vi "AM_PID_tester_2.vi"() -> ()   [LabVIEW 2013]
uses:
  DataMode.ctl
  Input_5782/5782_states.ctl
  <vilib>/Platform/TimedLoop/XDataNode/timing_clust.ctl
  <vilib>/Platform/TimedLoop/XDataNode/nitl_modes.ctl
  <vilib>/Platform/TimedLoop/XDataNode/wakeup.ctl
  <vilib>/rvi/FXPMathLib/FxpConvert/subVIs/nifxpmath_Convert_SimConfig.ctl
  <vilib>/fxp/LVFixedPointQuantizationPolicyTypeDef.ctl
  <vilib>/fxp/LVFixedPointOverflowPolicyTypeDef.ctl
  <vilib>/rvi/Emulation/niFpgaSctlEmulationGetInTimedLoop.vi
  <vilib>/rvi/Emulation/niFpgaEmulationReportErrorSimple.vi
  <vilib>/rvi/Emulation/niFpgaGetClockAttributes.vi
  <vilib>/rvi/eio/common/nirviEmuTemplateMethod_errors.vi
  <vilib>/rvi/Emulation/niFpgaCriticalErrorInLSC.vi
  <vilib>/rvi/DataTransferAndStorage/Register/Emulation/niFpgaRegisterEmulationFpgaImpl.vi
  <instcachedir>/0/niFpgaRegisterEmulationFpgaImpl_DCF4BC0110594B98B44A971D60CEEC4D.lvgen/niFpgaRegisterEmulationFpgaImpl_DCF4BC0110594B98B44A971D60CEEC4D_005.vi
  <vilib>/rvi/DataTransferAndStorage/Container/Common/niFpgaContainerGetUniqueNameForEmu.vi
  <instcachedir>/0/niFpgaRegisterEmulationFpgaImpl_DCF4BC0110594B98B44A971D60CEEC4D.lvgen/niFpgaRegisterEmulationFpgaImpl_DCF4BC0110594B98B44A971D60CEEC4D_016.vi
  <instcachedir>/0/niFpgaRegisterEmulationFpgaImpl_DCF4BC0110594B98B44A971D60CEEC4D.lvgen/niFpgaRegisterEmulationFpgaImpl_DCF4BC0110594B98B44A971D60CEEC4D_017.vi
  <instcachedir>/0/niFpgaRegisterEmulationFpgaImpl_DCF4BC0110594B98B44A971D60CEEC4D.lvgen/niFpgaRegisterEmulationFpgaImpl_DCF4BC0110594B98B44A971D60CEEC4D_012.vi
  <instcachedir>/0/niFpgaRegisterEmulationFpgaImpl_DCF4BC0110594B98B44A971D60CEEC4D.lvgen/niFpgaRegisterEmulationFpgaImpl_DCF4BC0110594B98B44A971D60CEEC4D_015.vi
  <vilib>/rvi/FIFO/Fifo_Resource/nirvififoEmulationReadFpgaImpl.vi
  <vilib>/rvi/interface/RandomDataEmulation/nirviRandomDataMultiElementFPGAFIFO.vi
  <instcachedir>/0/nirviRandomDataMultiElementFPGAFIFO_F2B80EDE0D7944A08478D8D26097D4DB.lvgen/nirviRandomDataMultiElementFPGAFIFO_F2B80EDE0D7944A08478D8D26097D4DB_005.vi
  <vilib>/rvi/interface/RandomDataEmulation/niFpgaRandomDataHandleErrors.vi
  <instcachedir>/0/niFpgaRegisterEmulationFpgaImpl_DCF4BC0110594B98B44A971D60CEEC4D.lvgen/niFpgaRegisterEmulationFpgaImpl_DCF4BC0110594B98B44A971D60CEEC4D_009.vi
  <vilib>/rvi/interface/RandomDataEmulation/nirviRandomDataFPGAFIFO.vi
  <vilib>/rvi/FXPMathLib/FxpConvert/simVIs/DllFxpConvertTemp_sub.vi
  <vilib>/rvi/FIFO/Fifo_Resource/nirvififoEmulationWriteFpgaImpl.vi
  <vilib>/Platform/TimedLoop/XDataNode/XDataNode.xnode
  <vilib>/eio/EIONode/EIONode.xnode
  <vilib>/rvi/DataTransferAndStorage/Container/XNode/niFpgaContainer.xnode
  <vilib>/rvi/DataTransferAndStorage/Register/Emulation/niFpgaRegisterEmulation.vi
  <vilib>/rvi/FIFO/Fifo_Resource/nirvififoEmulationRead.vi
  <vilib>/rvi/interface/RandomDataEmulation/nirviRandomDataFpgaMultiElementTemplate.vi
  <vilib>/rvi/interface/RandomDataEmulation/nirviRandomDataFpgaReadWriteTemplate.vi
  <vilib>/rvi/FXPMathLib/FxpInterpret/XNode/nifxpmath_Interpret.xnode
  <vilib>/rvi/FXPMathLib/FxpConvert/XNode/nifxpmath_Convert.xnode
  <vilib>/rvi/FIFO/Fifo_Resource/nirvififoEmulationWrite.vi
  <vilib>/rvi/FXPMathLib/FxpSub/XNode/nifxpmath_Sub.xnode
  <vilib>/Platform/TimedLoop/XDataNode/XDNodeRunTimeDep.lvlib
  <vilib>/rvi/FXPMathLib/sim/FxpSim.dll
panel:
  in  "AM phase":fxp<+,64,64>
  in  "Continuous":bool
  in  "Downsample":fxp<+,8,8>=1.0
  in  "new coeffs":bool
  in  "FIR coeffs":fxp<+/-,18,18>[](array[numeric])
  in  "CIC Gain":fxp<+/-,32,1>=0.00390625 format="%#_32g"
  in  "Acquisition running":bool
  in  "Phase output":fxp<+,64,64>[](array[numeric])=[0.0, 0.0, 0.0, 0.0, 0.0, 0.0, 0.0, 0.0]
  in  "Simulated phase 5782":fxp<+,64,64>[](array[numeric])=[0.0, 0.0]
  in  "Mode":T1
  in  "Phase 5782":fxp<+,64,64>[](array[numeric])=[0.0, 0.0]
  out "IO Module\\Trigger Input":bool
  in  "IO Module\\AO Data Sync":bool=TRUE
  in  "IO Module\\SPI Write Data":u16
  out "IO Module\\SPI Read Data":u8
  in  "IO Module\\SPI Read":bool
  in  "IO Module\\SPI Write":bool
  in  "IO Module\\SPI Address":u16
  in  "IO Module\\SPI Device":u8
  out "IO Module\\SPI Idle":bool
  in  "delay phase":fxp<+,64,64>
  in  "User Command Commit":bool
  in  "User Command":u8
  out "User Command Idle":bool
  out "User Command Status":u8
  in  "User Data 0":u8
  in  "User Data 1":u8
  out "PLL Locked":bool
  out "User Error":bool
  out "Configured?":bool
  in  "5782 record length":u16=4000 caption="Samples Per Trigger" min=1 step=1
  in  "Trigger Acquisition":bool
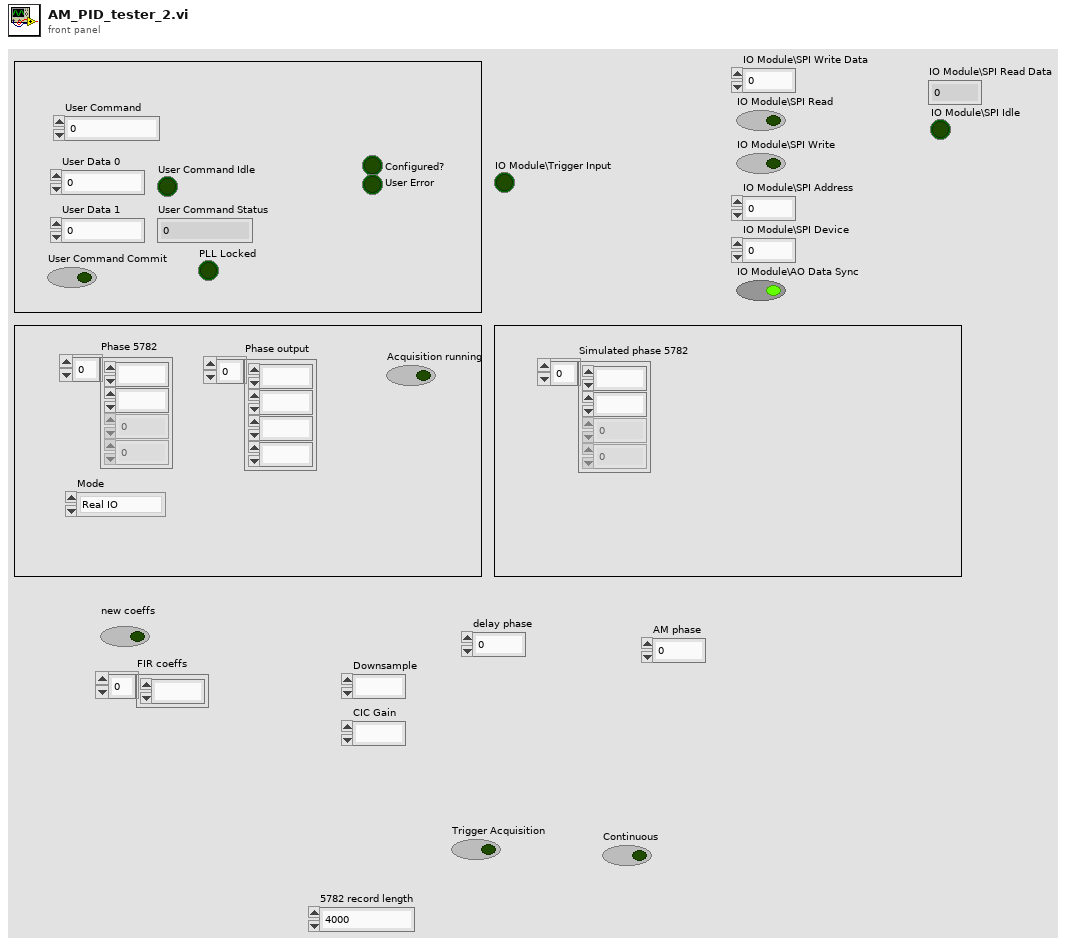
[diagram p1: front panel]
types:
  T1 = typedef "DataMode.ctl" = enum16{"Real IO", "Simulated"}
  T2 = typedef "5782_states.ctl" = enum8{"Wait for trigger", "Acquisition", "Send record length", "Quiet period"}
  T3 = typedef "XDNodeRunTimeDep.lvlib/timing_clust.ctl" = cluster{"Expected End [f-1]":u64, "Actual End [f-1]":u64, "Finished Late? [f-1]":bool, "Expected End [i-1]":u64, "Actual End [i-1]":u64, "Finished Late? [i-1]":bool, "Expected Start [i]":u64, "Actual Start [i]":u64, "Expected Start [f]":u64, "Actual Start [f]":u64, "Source Name":string, "Structure Name":string, "Period":i64, "Deadline":i64, "Offset":i64, "Start":i64, "Priority":i32, "Timeout":i32, "Mode":T4, "Wakeup Reason":T5, "Error":errorcluster, "Source Type":string, "Secondary Source Type":string, "Global End Time":u64, "Global Start Time":u64, "Frame Duration":u64, "Iteration Duration":u64, "Assigned CPU":i32, "I/O Scan Engine Mode":u32}
  T4 = typedef "XDNodeRunTimeDep.lvlib/nitl_modes.ctl" = enum32{"No Change", "Process missed periods, maintain original phase", "Discard missed periods, maintain original phase", "Process missed periods, ignore original phase", "Discard missed periods, ignore original phase"}
  T5 = typedef "XDNodeRunTimeDep.lvlib/wakeup.ctl" = enum32{"Normal", "Aborted", "Asynchronous wakeup", "Timing source error", "Timed loop error", "Timeout"}
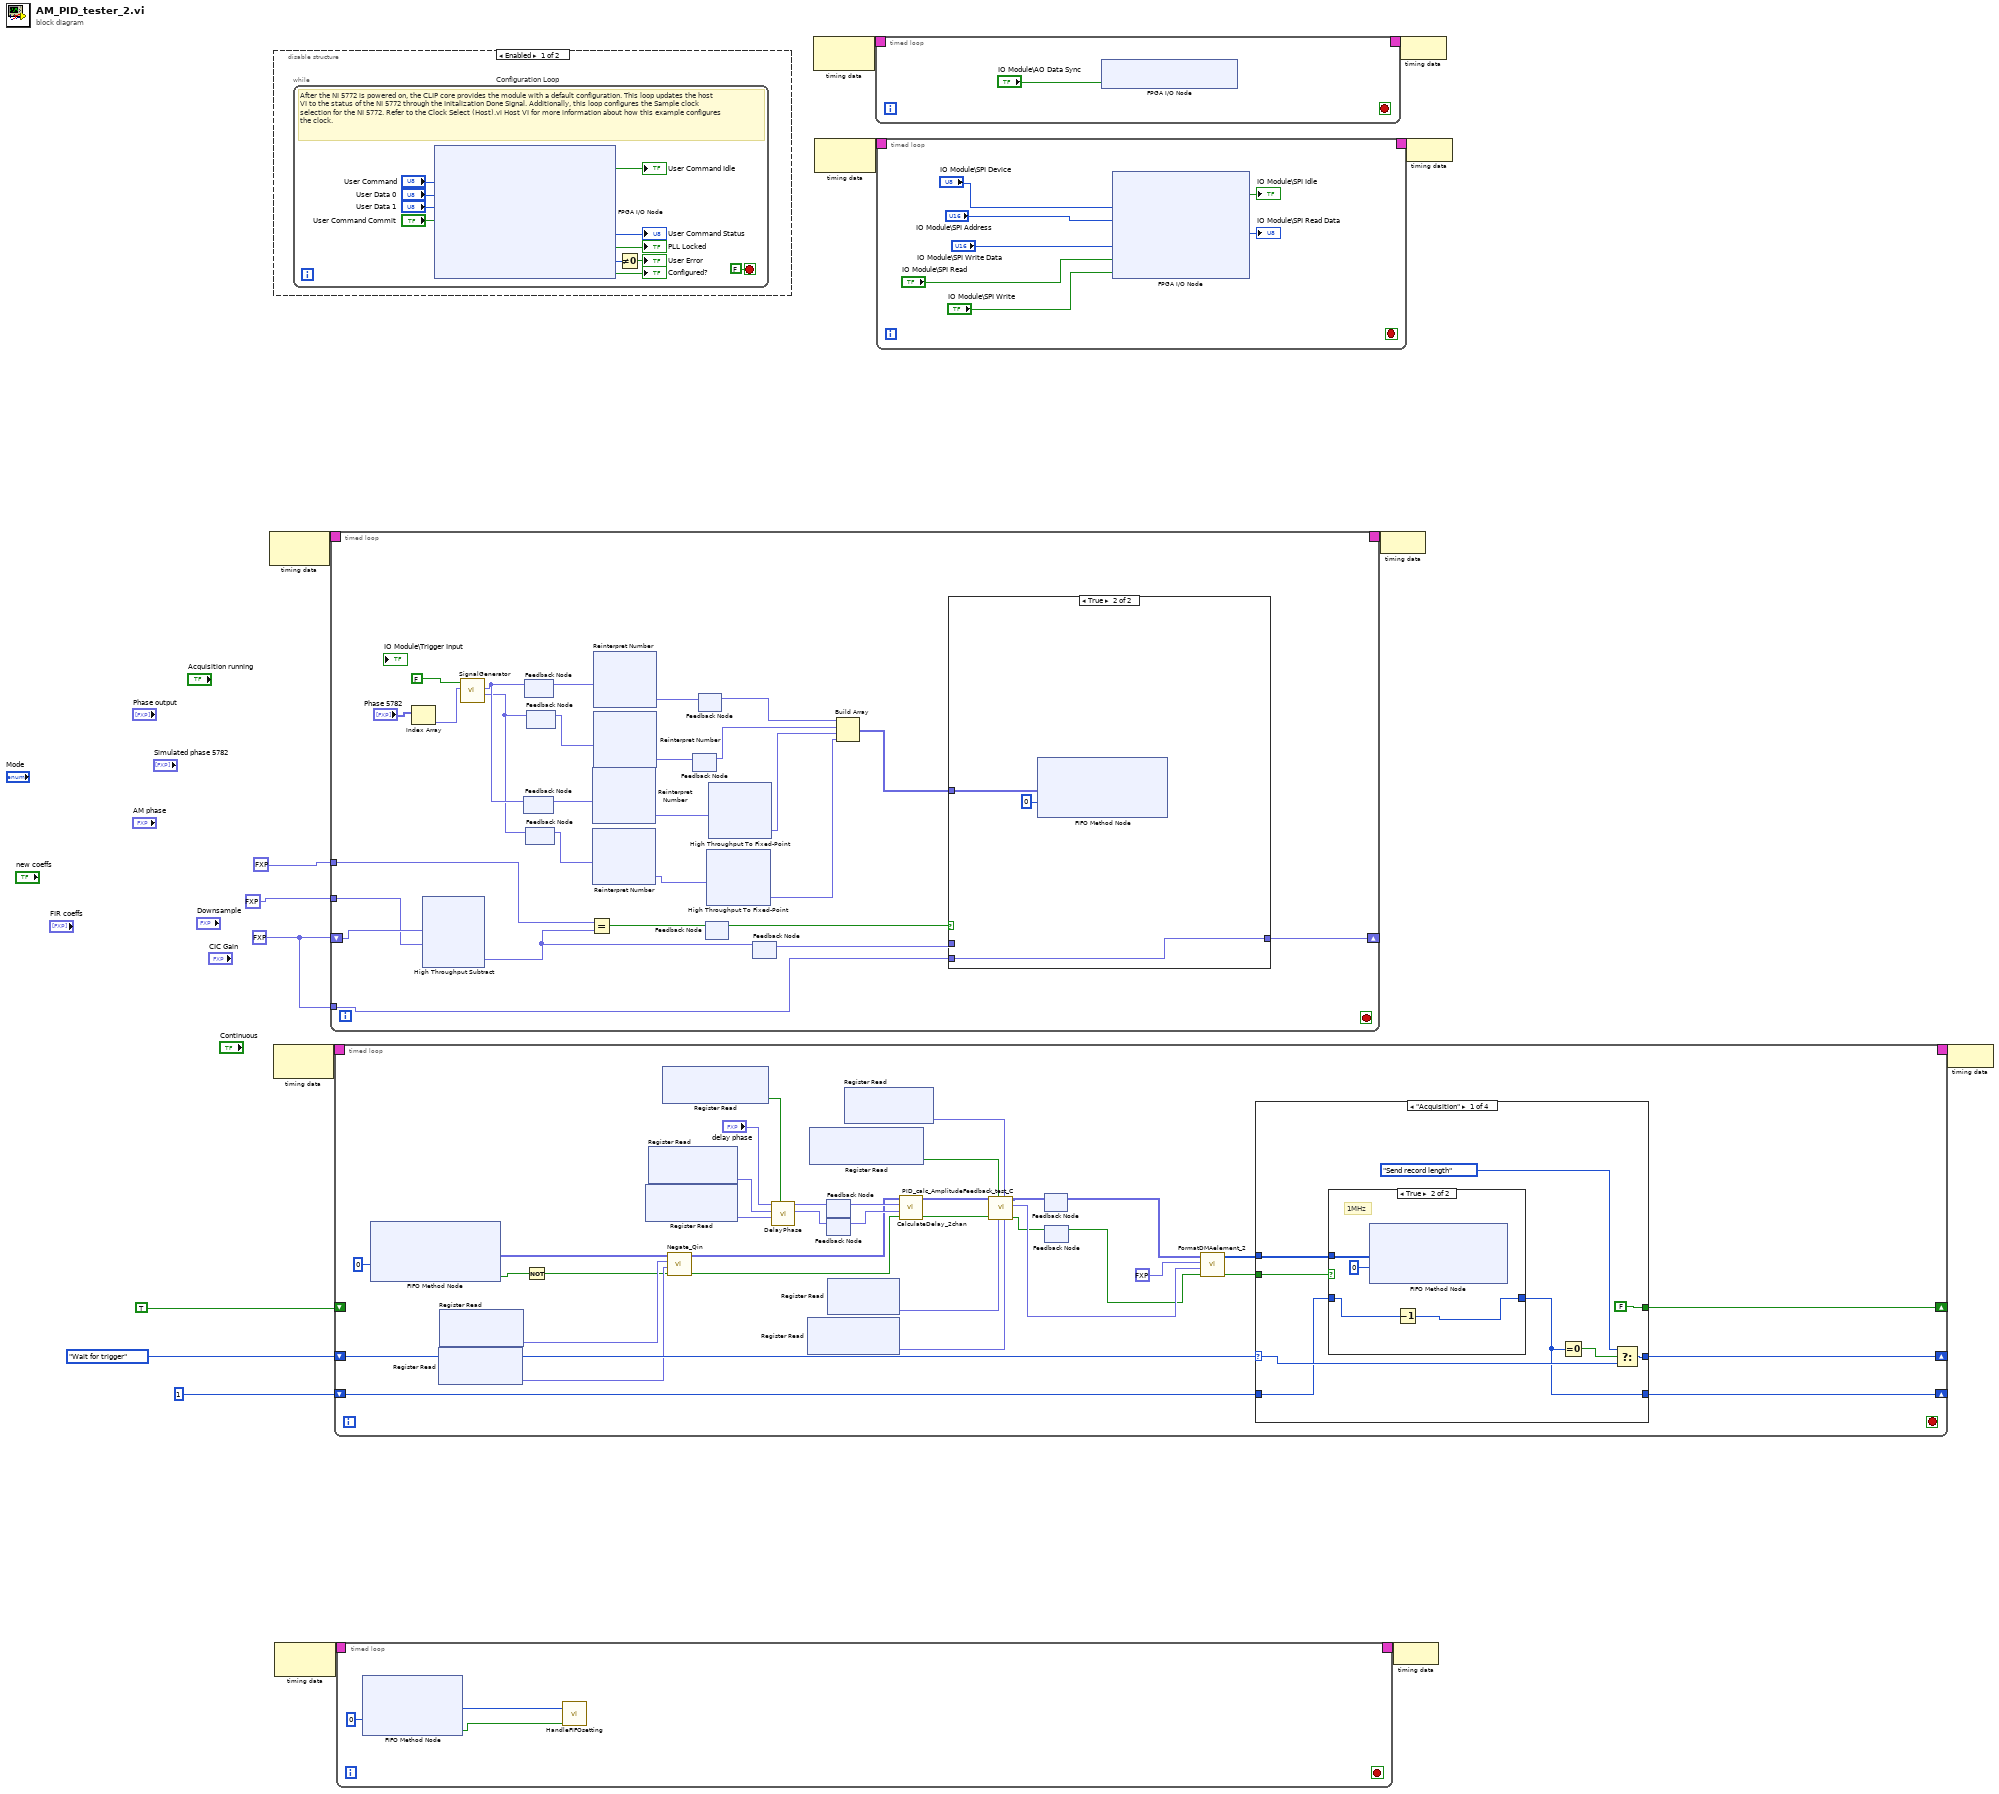
[diagram p0: block diagram]
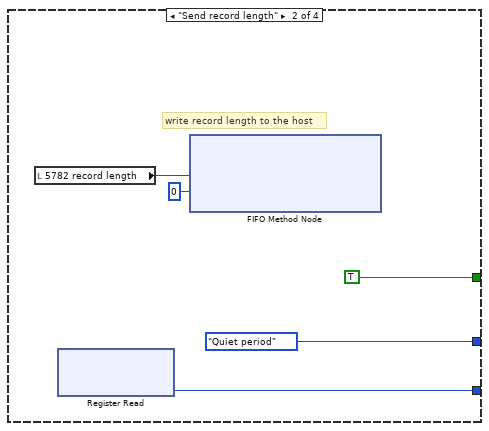
[diagram p4: hidden frame]
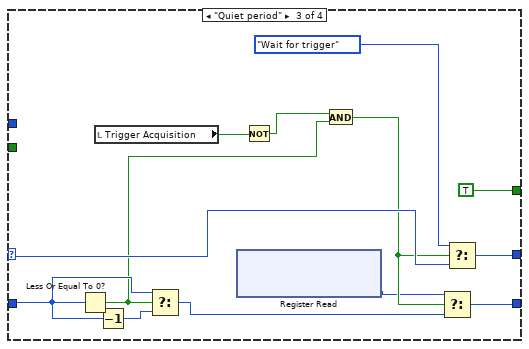
[diagram p5: hidden frame]
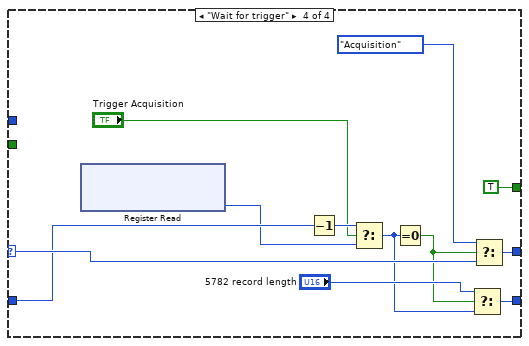
[diagram p6: hidden frame]
diagram:
  w3 = fxp<+/-,8,8> 5.0 ("x")
  n1 = node-c288() -> (w2:T3)  [unwired: 1 in]
  n2 = disable-structure shown="Enabled" {
    frame Enabled {
      n3 = while "Configuration Loop" {
        stop <- FALSE stop-if-true
        # "After the NI 5772 is powered on, the CLIP core provides the module with a default configuration. This loop updates the host VI to the status of the NI 5772 through the Initalization Done Signal. Additionally, this loop configures the Sample clock selection for the NI 5772. Refer to the Clock Select (Host).vi Host VI for more information about how this example configures the clock."
        n4 = xnode "FPGA I/O Node"("IO Module\\User Command"="User Command", "IO Module\\User Data 0"="User Data 0", "IO Module\\User Data 1"="User Data 1", "IO Module\\User Command Commit"="User Command Commit") -> ("IO Module\\User Command Idle"=→"User Command Idle":bool, "IO Module\\User Command Status"=→"User Command Status":u8, "IO Module\\PLL Locked"=→"PLL Locked":bool, "IO Module\\User Error"=w22:u8, "IO Module\\Initialization Done"=→"Configured?":bool)  [unwired: 9 in, 9 out]
        n5 = Not Equal To 0?(x=w22) -> (x != 0?=→"User Error":bool)
      }
    }
    frame Disabled {
    }
  }
  n6 = node-c288() -> (w16:T3)  [unwired: 1 in]
  n7 = node-c288() -> (w11:T3)  [unwired: 1 in]
  n8 = timed-loop {
    shift-right: [w50] -> _
    shift-left: w3 -> [w54]
    tunnel: fxp<+/-,8,8> 1.0 ("y") -> [w53]
    tunnel: fxp<+/-,8,8> 0.0 ("y") -> [w52]
    tunnel: w3 -> [w51]
    timing: w2 -> [_]
    timing-out: [_] -> w1
    stop <- _ stop-if-true
    n9 = Index Array(array="Phase 5782") -> (element=w28:fxp<+,64,64>)  [unwired: 1 in]
    n10 = xnode "High Throughput Subtract"("x"=w54, "y"=w53) -> ("x-y"=w47:fxp<+/-,8,8>)
    n11 = call "SignalGenerator.vi"("phase"=w28, "Reset"=FALSE) -> ("Cos"=w39:fxp<+/-,16,0>, "Sin"=w40:fxp<+/-,16,0>)  [unwired: 7 in, 1 out]
    n12 = feedback #1() -> (w41:fxp<+/-,16,0>)  [unwired: 1 in]
    n13 = feedback-in #1(w40) -> ()
    n14 = feedback #2() -> (w44:fxp<+/-,16,0>)  [unwired: 1 in]
    n15 = feedback-in #2(w40) -> ()
    n16 = feedback #3() -> (w42:fxp<+/-,16,0>)  [unwired: 1 in]
    n17 = feedback-in #3(w39) -> ()
    n18 = feedback #4() -> (w43:fxp<+/-,16,0>)  [unwired: 1 in]
    n19 = feedback-in #4(w39) -> ()
    n20 = Equal?(x=w52, y=w47) -> (x = y?=w49:bool)
    n21 = xnode "Reinterpret Number"("x"=w41) -> ("y"=w38:fxp<+/-,16,15>)
    n22 = xnode "Reinterpret Number"("x"=w42) -> ("y"=w37:fxp<+/-,16,15>)
    n23 = xnode "Reinterpret Number"("x"=w44) -> ("y"=w36:fxp<+/-,16,14>)
    n24 = xnode "Reinterpret Number"("x"=w43) -> ("y"=w35:fxp<+/-,16,14>)
    n25 = feedback #5() -> (w33:fxp<+/-,16,14>)  [unwired: 1 in]
    n26 = feedback-in #5(w35) -> ()
    n27 = feedback #6() -> (w34:fxp<+/-,16,14>)  [unwired: 1 in]
    n28 = feedback-in #6(w36) -> ()
    n29 = feedback #7() -> (w48:bool)  [unwired: 1 in]
    n30 = feedback-in #7(w49) -> ()
    n31 = xnode "High Throughput To Fixed-Point"("x"=w37) -> ("y"=w31:fxp<+/-,16,14>)
    n32 = xnode "High Throughput To Fixed-Point"("x"=w38) -> ("y"=w32:fxp<+/-,16,14>)
    n33 = feedback #8() -> (w46:fxp<+/-,8,8>)  [unwired: 1 in]
    n34 = feedback-in #8(w47) -> ()
    n35 = Build Array(w34, w33, w32, w31) -> (w30:fxp<+/-,16,14>[])
    n36 = case shown="True" w48 {
      tunnel: w51 -> [_ w102]
      tunnel: w46 -> [w99 _]
      tunnel: [w99 w102] -> w50
      tunnel: w30 -> [_ w100]
      frame False {
      }
      frame True {
        n37 = xnode ("FIFO Method Node")("Element"=w100, "Timeout"=0) -> ()  [unwired: 1 in, 2 out]
      }
    }
  }
  n38 = timed-loop {
    timing: w16 -> [_]
    timing-out: [_] -> w15
    shift-right: [w137] -> _
    shift-left: 5782_states."Wait for trigger" ("5782 states") -> [w139]
    shift-right: [w136] -> _
    shift-left: u16 1 ("trigger samples") -> [w138]
    shift-right: [w131] -> _
    shift-left: TRUE -> [_]
    stop <- _ stop-if-true
    n39 = xnode ("FIFO Method Node")("Timeout"=0) -> ("Element"=w113:fxp<+/-,16,14>[], "Timed Out?"=w134:bool)  [unwired: 1 in, 1 out]
    n40 = xnode ("Register Read")() -> ("Data"=w124:fxp<+/-,16,14>)  [unwired: 1 in, 1 out]
    n41 = xnode ("Register Read")() -> ("Data"=w125:fxp<+/-,16,14>)  [unwired: 1 in, 1 out]
    n42 = Not(x=w134) -> (.not. x?=w114:bool)
    n43 = xnode ("Register Read")() -> ("Data"=w121:fxp<+/-,16,0>)  [unwired: 1 in, 1 out]
    n44 = xnode ("Register Read")() -> ("Data"=w122:fxp<+/-,16,0>)  [unwired: 1 in, 1 out]
    n45 = xnode ("Register Read")() -> ("Data"=w123:bool)  [unwired: 1 in, 1 out]
    n46 = call "Negate_Qin.vi"("valid in"=w114, "DC offset chan 1"=w124, "DC offset chan 0"=w125, "Data in"=w113) -> ("valid out"=w110:bool, "Data out"=w111:fxp<+/-,16,14>[])  [unwired: 6 in]
    n47 = call "DelayPhase.vi"("Use fixed delay"=w123, "fixed cos_fi"=w121, "fixed sin fi"=w122, "delay phase"="delay phase") -> ("cos_fi"=w126:fxp<+/-,16,0>, "sin fi"=w127:fxp<+/-,16,0>)  [unwired: 6 in]
    n48 = xnode ("Register Read")() -> ("Data"=w116:fxp<+/-,32,6>)  [unwired: 1 in, 1 out]
    n49 = xnode ("Register Read")() -> ("Data"=w118:bool)  [unwired: 1 in, 1 out]
    n50 = feedback-in #9(w127) -> ()
    n51 = feedback #9() -> (w130:fxp<+/-,16,0>)  [unwired: 1 in]
    n52 = feedback #10() -> (w129:fxp<+/-,16,0>)  [unwired: 1 in]
    n53 = feedback-in #10(w126) -> ()
    n54 = xnode ("Register Read")() -> ("Data"=w117:fxp<+/-,32,6>)  [unwired: 1 in, 1 out]
    n55 = xnode ("Register Read")() -> ("Data"=w115:fxp<+/-,32,6>)  [unwired: 1 in, 1 out]
    n56 = call "CalculateDelay_2chan.vi"("input valid"=w110, "cos_fi"=w129, "sin fi"=w130, "Data in"=w111) -> ("output valid"=w119:bool, "Data out"=w120:fxp<+/-,16,14>[])  [unwired: 6 in]
    n57 = call "PID_calc_AmplitudeFeedback_test_C.vi"("Kd/Tau"=w116, "Ki*Tau"=w115, "Kp"=w117, "Enabled"=w118, "input valid"=w119, "Data in"=w120) -> ("output valid"=w107:bool, "c(t)"=w109:fxp<+/-,32,21>, "data out"=w112:fxp<+/-,16,14>[])  [unwired: 2 in, 1 out]
    n58 = feedback #11() -> (w106:fxp<+/-,16,14>[])  [unwired: 1 in]
    n59 = feedback-in #11(w112) -> ()
    n60 = feedback #12() -> (w105:bool)  [unwired: 1 in]
    n61 = feedback-in #12(w107) -> ()
    n62 = call "FormatDMAelement_2.vi"("valid in"=w105, "c(t) - AM"=w109, "c(t) - Phase"=fxp<+/-,32,4> 0.0, "Data in"=w106) -> ("valid out"=w132:bool, "Element"=w133:u64[])  [unwired: 6 in]
    n63 = case shown="\"Acquisition\"" w139 {
      selector: w139 -> [w148 _ w170 w183]
      tunnel: w138 -> [w144 _ w163 w174]
      tunnel: [w147 5782_states."Quiet period" ("5782 states") w169 w182] -> w137
      tunnel: [w141 w154 w171 w181] -> w136
      tunnel: w133 -> [w142 _ _ _]
      tunnel: w132 -> [w143 _ _ _]
      tunnel: [FALSE TRUE TRUE TRUE] -> w131
      frame "Acquisition" {
        n64 = case shown="True" w143 {
          tunnel: w142 -> [_ w153]
          tunnel: [w149 w150] -> w141
          tunnel: w144 -> [w149 w151]
          frame False {
          }
          frame True {
            # "1MHz"
            n65 = xnode ("FIFO Method Node")("Element"=w153, "Timeout"=0) -> ()  [unwired: 1 in, 2 out]
            n66 = Decrement(x=w151) -> (x-1=w150:u16)
          }
        }
        n67 = Equal To 0?(x=w141) -> (x = 0?=w145:bool)
        n68 = Select(t=5782_states."Send record length" ("5782 states"), s=w145, f=w148) -> (s? t:f=w147:T2)
      }
      frame "Send record length" {
        # "write record length to the host"
        n69 = local read "5782 record length"() -> (w155:u16)
        n70 = xnode ("Register Read")() -> ("Data"=w154:u16)  [unwired: 1 in, 1 out]
        n71 = xnode ("FIFO Method Node")("Element"=w155, "Timeout"=0) -> ()  [unwired: 1 in, 2 out]
      }
      frame "Quiet period" {
        n72 = Less Or Equal To 0?(x=w163) -> (x <= 0?=w162:bool)
        n73 = local read "Trigger Acquisition"() -> (w166:bool)
        n74 = Decrement(x=w163) -> (x-1=w164:u16)
        n75 = Select(t=w163, s=w162, f=w164) -> (s? t:f=w161:u16)
        n76 = xnode ("Register Read")() -> ("Data"=w160:u16)  [unwired: 1 in, 1 out]
        n77 = Not(x=w166) -> (.not. x?=w159:bool)
        n78 = And(x=w159, y=w162) -> (x .and. y?=w168:bool)
        n79 = Select(t=w160, s=w168, f=w161) -> (s? t:f=w171:u16)
        n80 = Select(t=5782_states."Wait for trigger" ("5782 states"), s=w168, f=w170) -> (s? t:f=w169:T2)
      }
      frame "Wait for trigger" {
        n81 = xnode ("Register Read")() -> ("Data"=w173:u16)  [unwired: 1 in, 1 out]
        n82 = Decrement(x=w174) -> (x-1=w175:u16)
        n83 = Select(t=w175, s="Trigger Acquisition", f=w173) -> (s? t:f=w176:u16)
        n84 = Equal To 0?(x=w176) -> (x = 0?=w177:bool)
        n85 = Select(t="5782 record length", s=w177, f=w176) -> (s? t:f=w181:u16)
        n86 = Select(t=5782_states."Acquisition" ("5782 states"), s=w177, f=w183) -> (s? t:f=w182:T2)
      }
    }
  }
  n87 = timed-loop {
    timing: w11 -> [_]
    timing-out: [_] -> w10
    stop <- _ stop-if-true
    n88 = xnode ("FIFO Method Node")("Timeout"=0) -> ("Element"=w187:u64, "Timed Out?"=w186:bool)  [unwired: 1 in, 1 out]
    n89 = call "HandleFIFOsetting.vi"("timed out"=w186, "Value"=w187) -> ()  [unwired: 10 in]
  }
  n90 = node-c288() -> (w7:T3)  [unwired: 1 in]
  n91 = node-c288() -> (w9:T3)  [unwired: 1 in]
  n92 = timed-loop {
    timing: w7 -> [_]
    timing-out: [_] -> w6
    stop <- _ stop-if-true
    n93 = xnode "FPGA I/O Node"("IO Module\\AO Data Sync"="IO Module\\AO Data Sync") -> ()  [unwired: 1 in, 1 out]
  }
  n94 = timed-loop {
    timing: w9 -> [_]
    timing-out: [_] -> w8
    stop <- _ stop-if-true
    n95 = xnode "FPGA I/O Node"("IO Module\\SPI Device"="IO Module\\SPI Device", "IO Module\\SPI Address"="IO Module\\SPI Address", "IO Module\\SPI Write Data"="IO Module\\SPI Write Data", "IO Module\\SPI Read"="IO Module\\SPI Read", "IO Module\\SPI Write"="IO Module\\SPI Write") -> ("IO Module\\SPI Idle"=→"IO Module\\SPI Idle":bool, "IO Module\\SPI Read Data"=→"IO Module\\SPI Read Data":u8)  [unwired: 7 in, 7 out]
  }
  n96 = node-c288(w1) -> ()
  n97 = node-c288(w10) -> ()
  n98 = node-c288(w6) -> ()
  n99 = node-c288(w8) -> ()
  n100 = node-c288(w15) -> ()
